vi "DAQ_2ch_sub.vi"() -> (0 "vol_out 2":dbl, 2 "vol_out":dbl)   [LabVIEW 2021]
panel:
  out "웨이브폼 그래프 2":dbl[](graph)
  out "웨이브폼 그래프":dbl[](graph)
  out "부분배열 2":dbl[](array[numeric])
  out "부분배열":dbl[](array[numeric])
  out "data 2":dynamicdata(graph) caption="data"
  in  "샘플 개수":i32=100
  in  "속도":dbl=1000.0
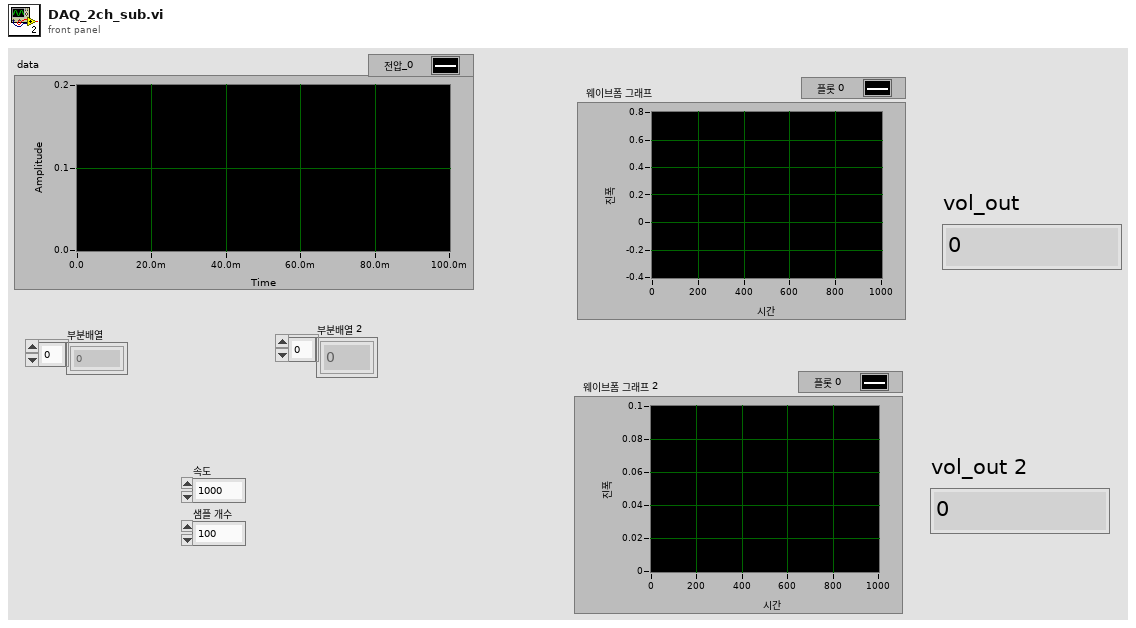
[diagram p1: front panel]
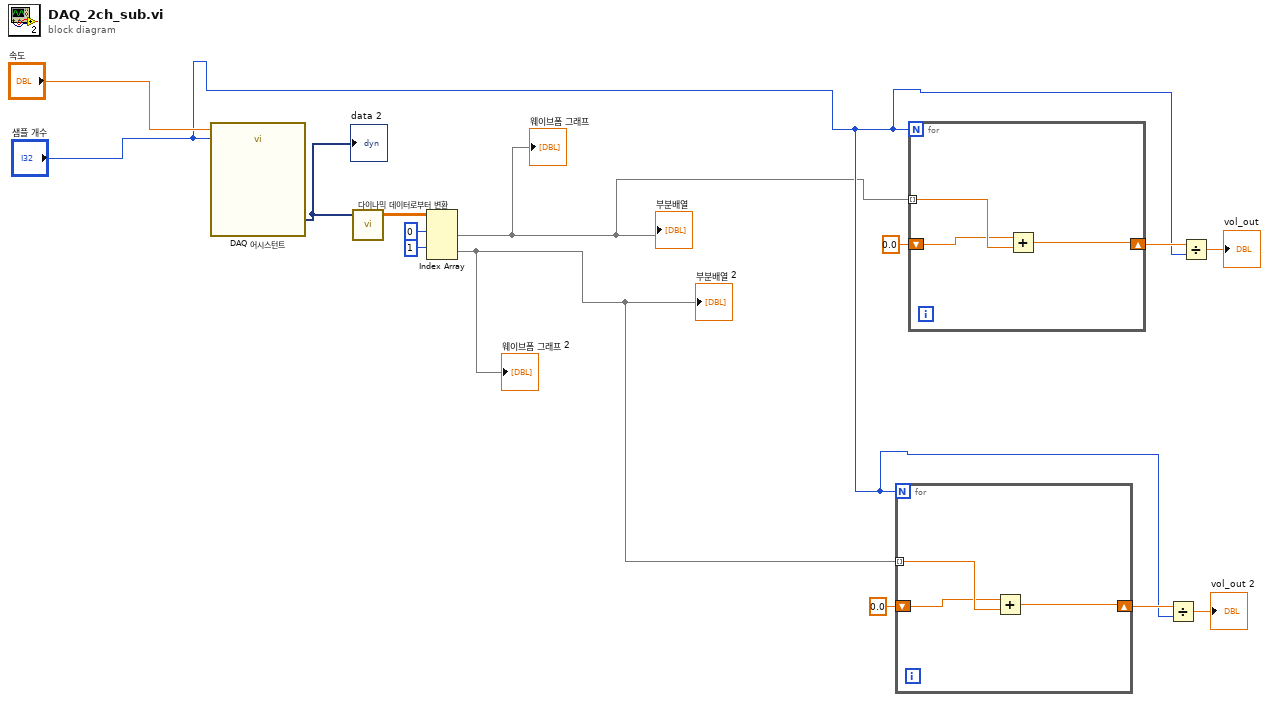
[diagram p0: block diagram]
diagram:
  n1 = call "DAQ 어시스턴트"("속도"="속도", "샘플 개수"="샘플 개수") -> ("data"=w13:dynamicdata)  [unwired: 15 in, 2 out]
  "data 2" <- w13
  n2 = call "다이나믹 데이터로부터 변환"("Dynamic Data Type"=w13) -> ("Array"=w12:dbl[][])  [unwired: 3 in]
  n3 = Index Array(array=w12, index (row) #1=0 ("인덱스 (행)"), index (row) #2=1 ("인덱스 (행)")) -> (element #1=w2:dbl[], element #2=w1:dbl[])  [unwired: 2 in]
  "부분배열" <- w2
  "부분배열 2" <- w1
  "웨이브폼 그래프 2" <- w1
  "웨이브폼 그래프" <- w2
  n4 = for {
    N: "샘플 개수" -> [_]
    tunnel: w1 -> [w17] mode=indexing
    shift-right: [w16] -> w5
    shift-left: 0.0 -> [w15]
    n5 = Add(x=w15, y=w17) -> (x+y=w16:dbl)
  }
  n6 = for {
    N: "샘플 개수" -> [_]
    tunnel: w2 -> [w20] mode=indexing
    shift-right: [w19] -> w8
    shift-left: 0.0 -> [w18]
    n7 = Add(x=w18, y=w20) -> (x+y=w19:dbl)
  }
  n8 = Divide(x=w5, y="샘플 개수") -> (x/y=→"vol_out 2":dbl)
  n9 = Divide(x=w8, y="샘플 개수") -> (x/y=→"vol_out":dbl)
